vi "Test PCAN-USB Read DBC Signals.vi"(11 "Test Case In":refnum<class "Test Communicator gRPC.lvclass">) -> (0 "error out":errorcluster, 3 "Test Case Out":refnum<class "Test Communicator gRPC.lvclass">)   [LabVIEW 2025, in "Test Communicator gRPC.lvclass"]
uses:
  Test Communicator gRPC.lvclass/Test Communicator gRPC.ctl
  Test Communicator gRPC.lvclass
  Source/Configure Strategies/PCAN-USB Strategies/PCAN-USB Read-Write Raw CAN Frame Strategy/PCAN Read-Write Raw CAN Frame Strategy.lvclass
  D:/git/HAL/HAL-Devices/Source/Configure Strategies/PCAN-USB Strategies/PCAN-USB Base Strategy/PCAN Base Strategy.lvclass
  D:/git/HAL/Source/Interfaces/IConfigure/IConfigure.lvclass
  D:/git/HAL/Source/Interfaces/IClose/IClose.lvclass
  D:/git/HAL/Source/Interfaces/IInitialize/IInitialize.lvclass
  D:/git/HAL/Source/Interfaces/ICommunicate/ICommunicate.lvclass
  D:/git/HAL/Source/Interfaces/IRunnable/IRunnable.lvclass
  D:/git/HAL/Source/Interfaces/IValidate Configuration/IValidate Configuration.lvclass
  D:/git/HAL/HAL-Devices/Source/Configure Strategies/PCAN-USB Strategies/PCAN-USB Read-Write Raw CAN Frame Strategy/PCAN Read-Write Raw CAN Frame Strategy.lvclass
  C:/Program Files/National Instruments/LabVIEW 2025/vi.lib/Astemes/LUnit/Test Case.lvclass
  C:/Program Files/National Instruments/LabVIEW 2025/vi.lib/Astemes/LUnit/LUnit Runnable.lvclass
  D:/git/HAL/HAL-Devices/Tests/New folder/Test Communicator gRPC.lvclass
  <vilib>/Astemes/LUnit/Test Case.lvclass
  Source/DBC Communicator/DBC Communicator.lvclass
panel:
  out "Time Stamp":timestamp format="%<%x %.3X>T"
  out "Array":dbl[](array[numeric])
  out "Value":dbl
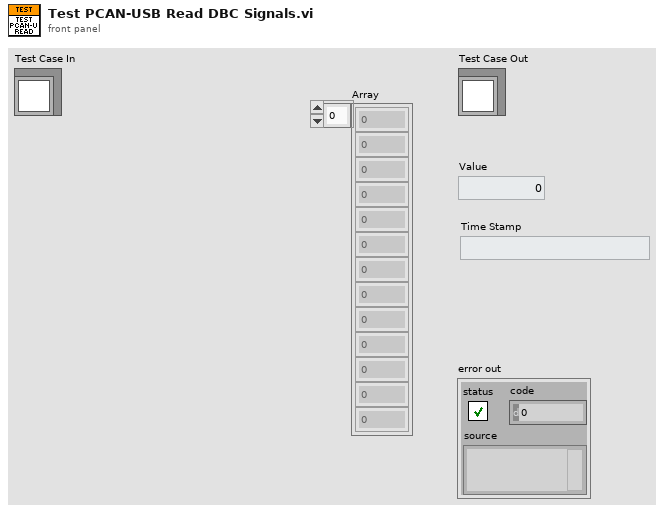
[diagram p1: front panel]
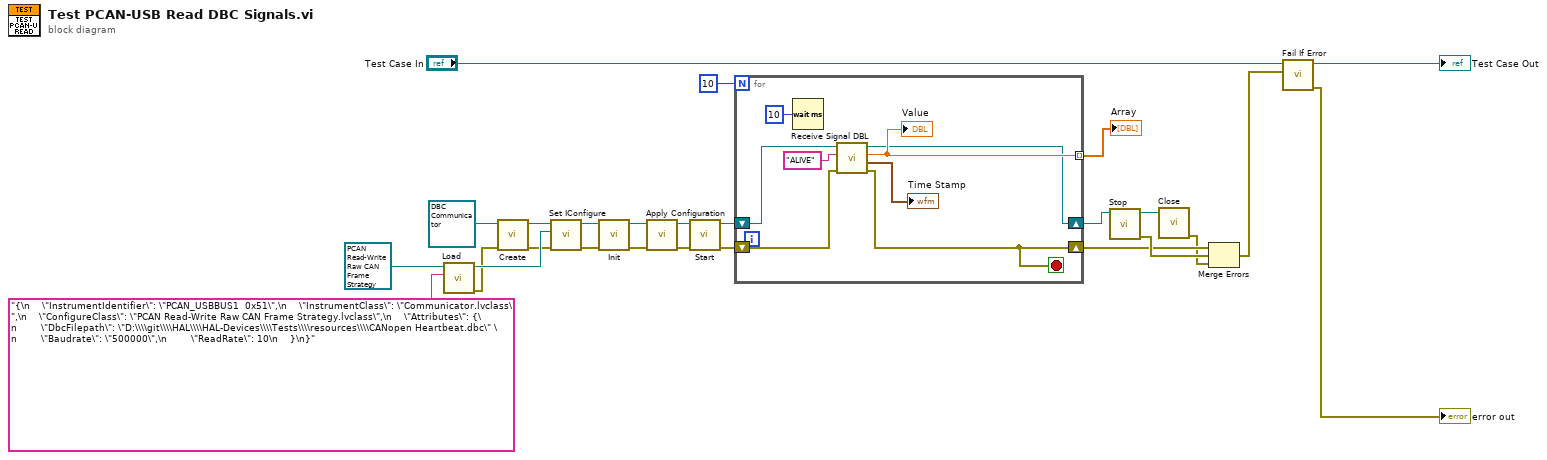
[diagram p0: block diagram]
diagram:
  n1 = call-dynamic "Load.vi"("Source"="{\n    \"InstrumentIdentifier\": \"PCAN_USBBUS1  0x51\",\n    \"InstrumentClass\": \"Communicator.lvclass\",\n    \"ConfigureClass\": \"PCAN Read-Write Raw CAN Frame Strategy.lvclass\",\n    \"Attributes\": {\n        \"DbcFilepath\": \"D:\\\\git\\\\HAL\\\\HAL-Devices\\\\Tests\\\\resources\\\\CANopen Heartbeat.dbc\" \n        \"Baudrate\": \"500000\",\n        \"ReadRate\": 10\n    }\n}", "PCAN-USB Read-Write Raw CAN Frame Strategy in"=refnum<class "PCAN Read-Write Raw CAN Frame Strategy.lvclass"> refnum ("PCAN-USB Read-Write Raw CAN Frame Strategy")) -> ("error out"=w8:errorcluster, "PCAN-USB Read-Write Raw CAN Frame Strategy out"=w23:refnum<class "PCAN Read-Write Raw CAN Frame Strategy.lvclass">)  [unwired: 8 in]
  n2 = call-dynamic "Create.vi"("Error In"=w8, "reference in"=refnum<class "DBC Communicator.lvclass"> refnum ("NI9862 in")) -> ("Error Out"=w1:errorcluster, "reference out"=w2:refnum<class "DBC Communicator.lvclass">)  [unwired: 8 in]
  n3 = call-dynamic "Set IConfigure.vi"("Error In"=w1, "IConfigure"=w23, "Communicator in"=w2) -> ("Error Out"=w22:errorcluster, "Communicator out"=w21:refnum<class "DBC Communicator.lvclass">)  [unwired: 7 in]
  n4 = call-dynamic "Init.vi"("Error In"=w22, "Communicator in"=w21) -> ("Error Out"=w20:errorcluster, "Communicator out"=w19:refnum<class "DBC Communicator.lvclass">)  [unwired: 8 in]
  n5 = call-dynamic "Apply Configuration.vi"("Error In"=w20, "reference in"=w19) -> ("Error Out"=w12:errorcluster, "reference out"=w13:refnum<class "DBC Communicator.lvclass">)  [unwired: 8 in]
  n6 = call-dynamic "Start.vi"("Error In"=w12, "Communicator in"=w13) -> ("Error Out"=w16:errorcluster, "Communicator out"=w17:refnum<class "DBC Communicator.lvclass">)  [unwired: 8 in]
  n7 = for {
    N: 10 -> [_]
    shift-right: [w27] -> w15
    shift-left: w17 -> [w28]
    shift-right: [w31] -> w9
    shift-left: w16 -> [w32]
    tunnel: [w30] -> w4 mode=indexing
    stop <- w31 stop-if-true
    n8 = Wait (ms)(milliseconds to wait=u32 10) -> ()  [unwired: 1 out]
    n9 = call "Receive Signal DBL.vi"("error in"=w32, "Signal Name"="ALIVE", "DBC Communication in"=w28) -> ("error out"=w31:errorcluster, "Time Stamp"=→"Time Stamp":timestamp, "Value"=w30:dbl, "DBC Communication out"=w27:refnum<class "DBC Communicator.lvclass">)  [unwired: 5 in]
    "Value" <- w30
  }
  "Array" <- w4
  n10 = call-dynamic "Stop.vi"("Communicator in"=w15) -> ("Error Out"=w10:errorcluster, "Communicator out"=w14:refnum<class "DBC Communicator.lvclass">)  [unwired: 9 in]
  n11 = call-dynamic "Close.vi"("reference in"=w14) -> ("Error Out"=w3:errorcluster)  [unwired: 9 in, 1 out]
  n12 = Merge Errors(w9, w10, w3) -> (w11:errorcluster)
  n13 = call <vilib>:"Fail If Error.vi"("Assert error"=w11, "LUnit Test Case In"="Test Case In") -> ("error out"=→"error out":errorcluster, "LUnit Test Case Out"=→"Test Case Out":refnum<class "Test Communicator gRPC.lvclass">)  [unwired: 8 in]
